vi "Boolean Array To U64 Array.vi"(5 "data in":bool[](array[boolean])) -> (6 "data out":u64[](array[numeric]))   [LabVIEW 2019]
uses:
  <instrlib>/_niInstr/Basic Elements/v1/FPGA/niInstr Basic Elements v1 FPGA.lvlib
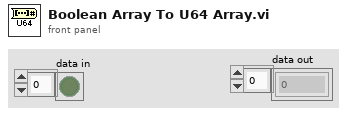
[diagram p1: front panel]
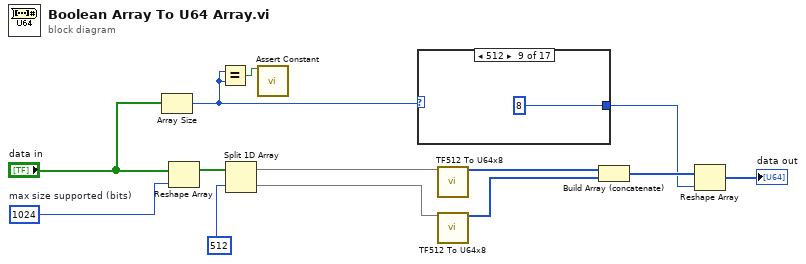
[diagram p0: block diagram]
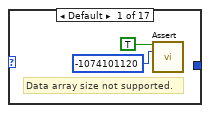
[diagram p2: hidden frame]
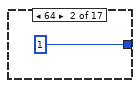
[diagram p3: hidden frame]
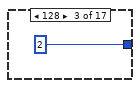
[diagram p4: hidden frame]
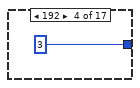
[diagram p5: hidden frame]
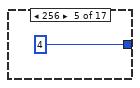
[diagram p6: hidden frame]
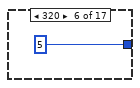
[diagram p7: hidden frame]
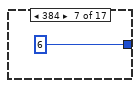
[diagram p8: hidden frame]
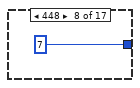
[diagram p9: hidden frame]
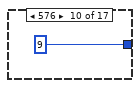
[diagram p10: hidden frame]
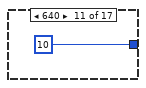
[diagram p11: hidden frame]
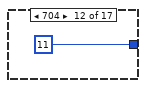
[diagram p12: hidden frame]
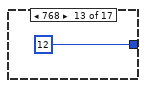
[diagram p13: hidden frame]
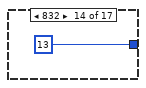
[diagram p14: hidden frame]
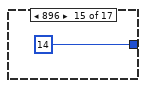
[diagram p15: hidden frame]
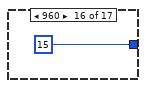
[diagram p16: hidden frame]
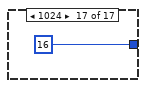
[diagram p17: hidden frame]
diagram:
  w13 = 1024  # max size supported (bits)
  n1 = Array Size(array="data in") -> (size(s)=w5:i32)
  n2 = Reshape Array("data in", w13) -> (w12:bool[])
  n3 = Equal?(x=w5, y=w5) -> (x = y?=w6:bool)
  n4 = Split 1D Array(array=w12, index=512) -> (first subarray=w4:bool[], second subarray=w3:bool[])
  n5 = call <instrlib>:"Assert Constant.vi"("constant terminal"=w6) -> ()  [unwired: 15 in]
  n6 = case shown="512" w5 {
    tunnel: [_ 1 2 3 4 5 6 7 8 9 10 11 12 13 14 15 16] -> w7
    frame Default {
      # "Data array size not supported."
      n7 = call <instrlib>:"Assert.vi"("assert"=TRUE, "error code"=-1074101120) -> ()  [unwired: 14 in]
    }
    frame 64 {
    }
    frame 128 {
    }
    frame 192 {
    }
    frame 256 {
    }
    frame 320 {
    }
    frame 384 {
    }
    frame 448 {
    }
    frame 512 {
    }
    frame 576 {
    }
    frame 640 {
    }
    frame 704 {
    }
    frame 768 {
    }
    frame 832 {
    }
    frame 896 {
    }
    frame 960 {
    }
    frame 1024 {
    }
  }
  n8 = call "TF512 To U64x8.vi"("data in"=w4) -> ("data out"=w1:u64[])  [unwired: 14 in]
  n9 = call "TF512 To U64x8.vi"("data in"=w3) -> ("data out"=w2:u64[])  [unwired: 14 in]
  n10 = Build Array (concatenate)(w1, w2) -> (w11:u64[])
  n11 = Reshape Array(w11, w7) -> (→"data out":u64[])
